vi "Read Requestor.vi"(8 "error in (no error)":errorcluster, 11 "Message with Names in":refnum<class "Message with Names.lvclass">) -> (0 "error out":errorcluster, 2 "Requestor":string, 3 "Message with Names out":refnum<class "Message with Names.lvclass">)   [LabVIEW 2015, in "Message with Names.lvclass"]
uses:
  Message with Names.lvclass
  Message with Names.lvclass/Message with Names.ctl
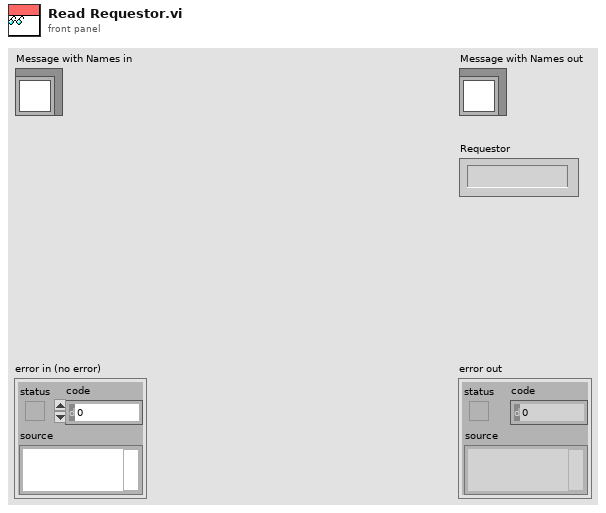
[diagram p1: front panel]
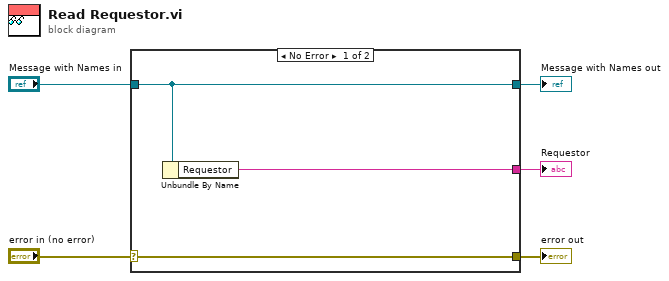
[diagram p0: block diagram]
diagram:
  n1 = case shown="No Error" "error in (no error)" {
    selector: "error in (no error)" -> [w8 w9]
    tunnel: [w8 w9] -> w4
    tunnel: [w7 w10] -> w2
    tunnel: "Message with Names in" -> [w7 w10]
    tunnel: [w6 _] -> w1
    frame No Error {
      n2 = Unbundle By Name(w7) -> ("Requestor"=w6:string)
    }
    frame Error {
    }
  }
  "error out" <- w4
  "Message with Names out" <- w2
  "Requestor" <- w1
